vi "Rapid Read_Alazar_Done.vi"(0 "DeviceIn":i32, 5 "Motion Board ID":T2=1 min=1 max=32 step=1, 7 "Motion System":T1=enum."NI 735x", 9 "SMAC Axis":u16, 11 "error out":errorcluster, 14 "Pause?":bool) -> (6 "Reverse?":bool, 15 "error out":errorcluster)   [LabVIEW 2022 SP3]
uses:
  <vilib>/Platform/TimedLoop/XDataNode/XDataNode.xnode
  <vilib>/Platform/TimedLoop/XDataNode/nitl_modes.ctl
  <vilib>/Platform/TimedLoop/XDataNode/XDNodeRunTimeDep.lvlib
  <vilib>/Platform/TimedLoop/XDataNode/wakeup.ctl
  <vilib>/Platform/TimedLoop/XDataNode/timing_clust.ctl
  Motion Controllers/NI_controller/-NI_MotionRoutines/MotionSys.ctl
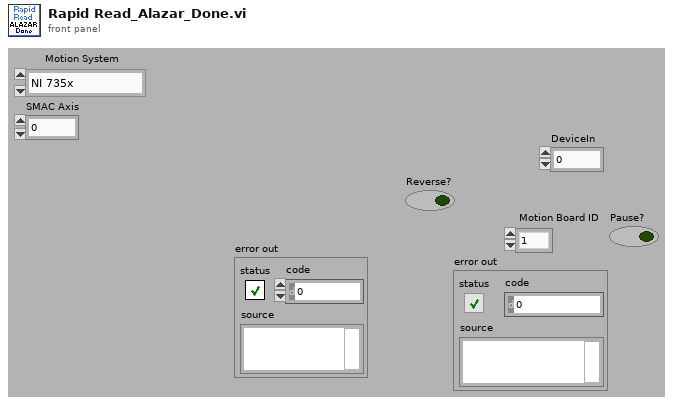
[diagram p1: front panel]
types:
  T1 = typedef "MotionSys.ctl" = enum16{"MM3000", "NI 735x", "Newport ESP", "No Motion Card", "Galil"}
  T2 = typedef "Board Id" = u8
  T3 = typedef "XDNodeRunTimeDep.lvlib/timing_clust.ctl" = cluster{"Expected End [f-1]":u64, "Actual End [f-1]":u64, "Finished Late? [f-1]":bool, "Expected End [i-1]":u64, "Actual End [i-1]":u64, "Finished Late? [i-1]":bool, "Expected Start [i]":u64, "Actual Start [i]":u64, "Expected Start [f]":u64, "Actual Start [f]":u64, "Source Name":string, "Structure Name":string, "Period":i64, "Deadline":i64, "Offset":i64, "Start":i64, "Priority":i32, "Timeout":i32, "Mode":T4, "Wakeup Reason":T5, "Error":errorcluster, "Source Type":string, "Secondary Source Type":string, "Global End Time":u64, "Global Start Time":u64, "Frame Duration":u64, "Iteration Duration":u64, "Assigned CPU":i32, "I/O Scan Engine Mode":u32}
  T4 = typedef "XDNodeRunTimeDep.lvlib/nitl_modes.ctl" = enum32{"No Change", "Process missed periods, maintain original phase", "Discard missed periods, maintain original phase", "Process missed periods, ignore original phase", "Discard missed periods, ignore original phase"}
  T5 = typedef "XDNodeRunTimeDep.lvlib/wakeup.ctl" = enum32{"Normal", "Aborted", "Asynchronous wakeup", "Timing source error", "Timed loop error", "Timeout"}
  T6 = typedef "Var" = u8
  T7 = cluster{"Run/Stop":bool, "Profile Complete":bool, "Motor Off ":bool, "Following Error":bool, "Limit Switch":bool, "Home Switch":bool, "SW Limit Switch":bool, "Watchdog":bool, "Velocity Threshold":bool, "Position Brkpt":bool, "Home Found":bool, "Index Found":bool, "High Speed Capture":bool, "Reverse Direction":bool, "Blend Complete":bool, "Move Complete":bool}
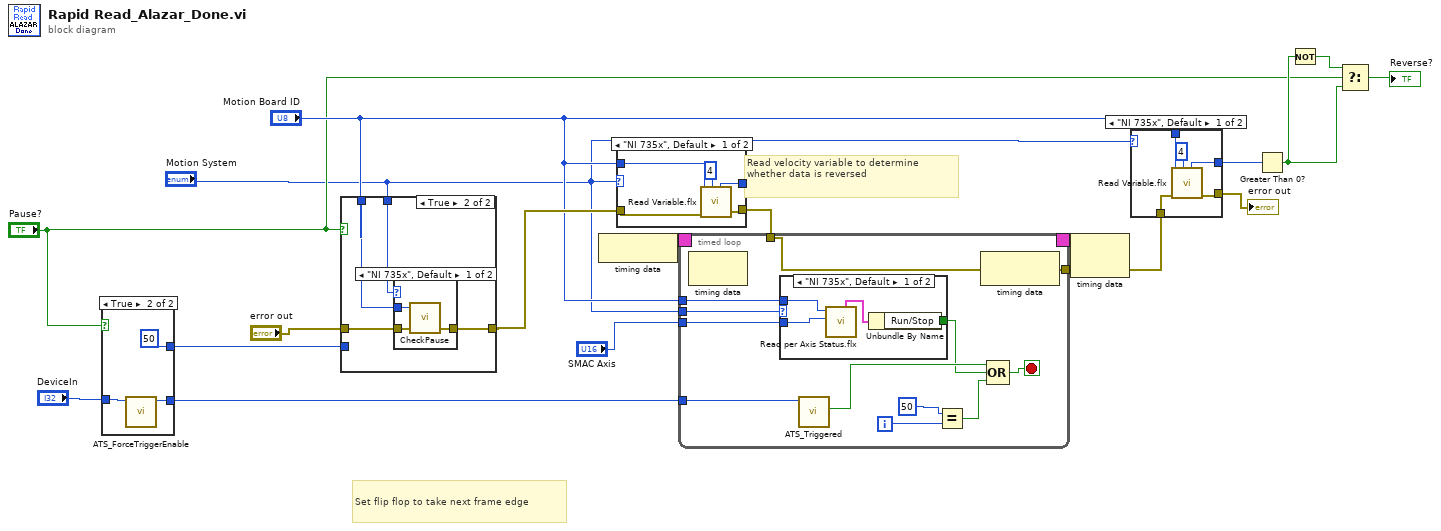
[diagram p0: block diagram]
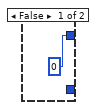
[diagram p2: hidden frame]
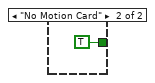
[diagram p3: hidden frame]
diagram:
  # "Set flip flop to take next frame edge"
  # "Read velocity variable to determine whether data is reversed"
  n1 = case shown="True" "Pause?" {
    tunnel: [_ w22] -> w11
    tunnel: "DeviceIn" -> [_ w21]
    tunnel: [u32 0 ("milliseconds to wait") u32 50 ("milliseconds to wait")] -> w4
    frame False {
    }
    frame True {
      n2 = call "ATS_ForceTriggerEnable.vi"("DeviceIn"=w21) -> ("DeviceOut"=w22:i32)  [unwired: 9 in, 1 out]
    }
  }
  n3 = case shown="True" "Pause?" {
    tunnel: [w23 w27] -> w13
    tunnel: "Motion Board ID" -> [_ w26]
    tunnel: "error out" -> [w23 w25]
    tunnel: w4 -> [_ _]
    tunnel: "Motion System" -> [_ w24]
    frame False {
    }
    frame True {
      n4 = case shown="\"NI 735x\", Default" w24 {
        tunnel: [w30 w31] -> w27
        tunnel: w26 -> [w29 _]
        tunnel: w25 -> [w28 w31]
        frame "NI 735x", Default {
          n5 = call "CheckPause.vi"("error in"=w28, "Motion Board ID"=w29) -> ("error out"=w30:errorcluster)  [unwired: 3 in]
        }
        frame "No Motion Card" {
        }
      }
    }
  }
  n6 = node-c288() -> (w15:T3)
  n7 = case shown="\"NI 735x\", Default" "Motion System" {
    tunnel: [w35 w37] -> w17
    tunnel: "Motion Board ID" -> [w34 _]
    tunnel: [w33 _] -> _
    tunnel: w13 -> [w32 w37]
    frame "NI 735x", Default {
      n8 = call <vilib>:"Read Variable.flx"("Var"=T6 4, "error in (no error)"=w32, "Board ID"=w34) -> ("error out"=w35:errorcluster, "Output"=w33:i32)  [unwired: 1 in, 4 out]
    }
    frame "No Motion Card" {
    }
  }
  n9 = timed-loop {
    tunnel: w17 -> [w48]
    tunnel: [w48] -> w18
    timing: w15 -> [_]
    timing-out: [_] -> w14
    tunnel: "Motion Board ID" -> [w43]
    tunnel: w11 -> [w42]
    tunnel: "SMAC Axis" -> [w40]
    tunnel: "Motion System" -> [w39]
    i -> [w47]
    stop <- w46 stop-if-true
    n10 = node-c288() -> ()  [unwired: 1 in, 1 out]
    n11 = case shown="\"NI 735x\", Default" w39 {
      tunnel: w43 -> [w52 _]
      tunnel: w40 -> [w51 _]
      tunnel: [w49 TRUE ("Run/Stop")] -> w38
      frame "NI 735x", Default {
        n12 = call <vilib>:"Read per Axis Status.flx"("Axis"=w51, "Board ID"=w52) -> ("Per Axis H/W Status"=w50:T7)  [unwired: 4 in, 3 out]
        n13 = Unbundle By Name(w50) -> ("Run/Stop"=w49:bool)
      }
      frame "No Motion Card" {
      }
    }
    n14 = call "ATS_Triggered.vi"("DeviceIn"=w42) -> ("Triggered"=w41:bool)  [unwired: 9 in, 1 out]
    n15 = Equal?(x=50, y=w47) -> (x = y?=w44:bool)
    n16 = node-c288() -> ()  [unwired: 1 in, 1 out]
    n17 = Compound Arithmetic op=OR(w41, w38, w44) -> (w46:bool)
  }
  n18 = node-c288(w14) -> ()  [unwired: 1 out]
  n19 = case shown="\"NI 735x\", Default" "Motion System" {
    tunnel: w18 -> [w59 w61]
    tunnel: [w58 w61] -> w8
    tunnel: "Motion Board ID" -> [w57 _]
    tunnel: [w56 _] -> w3
    frame "NI 735x", Default {
      n20 = call <vilib>:"Read Variable.flx"("Var"=T6 4, "error in (no error)"=w59, "Board ID"=w57) -> ("error out"=w58:errorcluster, "Output"=w56:i32)  [unwired: 1 in, 4 out]
    }
    frame "No Motion Card" {
    }
  }
  "error out" <- w8
  n21 = Greater Than 0?(x=w3) -> (x > 0?=w7:bool)
  n22 = Not(x=w7) -> (.not. x?=w5:bool)
  n23 = Select(t=w5, s="Pause?", f=w7) -> (s? t:f=→"Reverse?":bool)
